vi "Ciclo while_suma150_contador.vi"() -> ()   [LabVIEW 2013]
panel:
  out "SUMA150":dbl
  out "Contador":dbl
  out "Velocidad Promedio":dbl
  out "Velocidad":dbl(knob) scale=0.0..220.0
  # "GENERAR 10 PRUEBA DE VELOCIDAD\nLUEGO SUMAR LAS VELOCIDADES \nMAYORES A 150 Y OBTENER SU PROMEDIO"
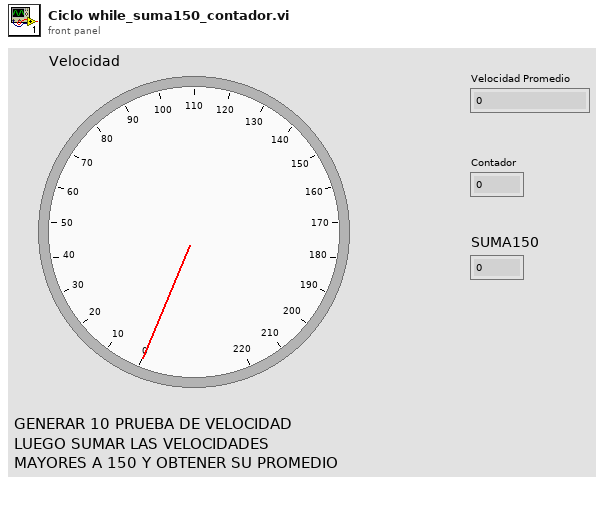
[diagram p1: front panel]
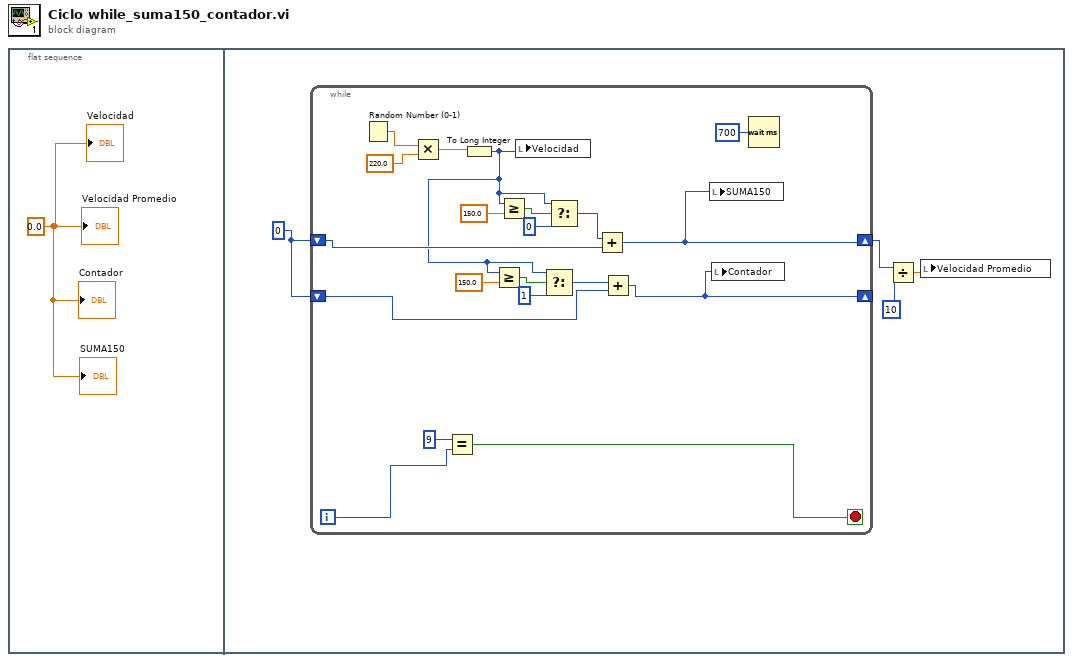
[diagram p0: block diagram]
diagram:
  n1 = flat-sequence {
    frame #0 {
      w1 = 0.0 ("Velocidad Promedio")
      "Velocidad" <- w1
      "Velocidad Promedio" <- w1
      "Contador" <- w1
      "SUMA150" <- w1
    }
    frame #1 {
      w5 = 0 ("x")
      n2 = while {
        shift-right: [w7] -> w4
        shift-left: w5 -> [w16]
        shift-right: [w9] -> _
        shift-left: w5 -> [w10]
        i -> [w25]
        stop <- w23 stop-if-true
        n3 = Random Number (0-1)() -> (number: 0 to 1=w22:dbl)
        n4 = Multiply(x=w22, y=220.0) -> (x*y=w20:dbl)
        n5 = Equal?(x=9, y=w25) -> (x = y?=w23:bool)
        n6 = To Long Integer(number=w20) -> (32bit integer=w8:i32)
        n7 = Greater Or Equal?(x=w8, y=150.0) -> (x >= y?=w13:bool)
        n8 = Greater Or Equal?(x=w8, y=150.0) -> (x >= y?=w18:bool)
        n9 = local write "Velocidad"(w8) -> ()
        n10 = Select(t=w8, s=w13, f=1) -> (s? t:f=w11:i32)
        n11 = Select(t=w8, s=w18, f=0) -> (s? t:f=w17:i32)
        n12 = Add(x=w17, y=w16) -> (x+y=w7:i32)
        n13 = Add(x=w11, y=w10) -> (x+y=w9:i32)
        n14 = local write "SUMA150"(w7) -> ()
        n15 = local write "Contador"(w9) -> ()
        n16 = Wait (ms)(milliseconds to wait=u32 700) -> ()  [unwired: 1 out]
      }
      n17 = Divide(x=w4, y=10) -> (x/y=w3:dbl)
      n18 = local write "Velocidad Promedio"(w3) -> ()
    }
  }
